vi "WriteOVABinFile.vi"(8 "error in (no error)":errorcluster, 10 "Matrix Selection":u8(ring) items=["A", "B", "C"], 11 "Measurement Data File Path":path) -> (0 "error out":errorcluster)   [LabVIEW 2012]
uses:
  bin/OVA32.dll
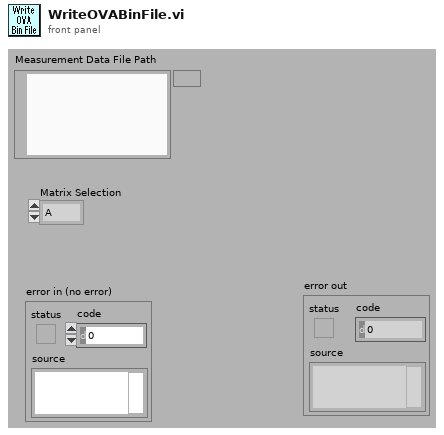
[diagram p1: front panel]
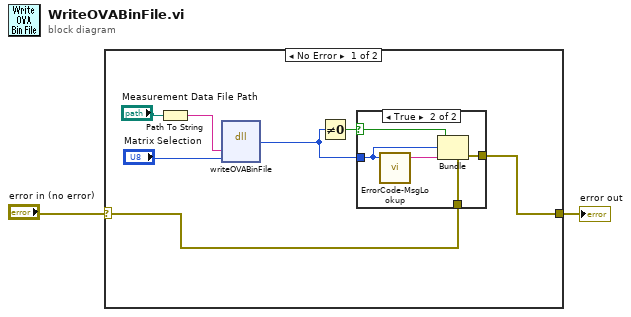
[diagram p0: block diagram]
diagram:
  n1 = case shown="No Error" "error in (no error)" {
    selector: "error in (no error)" -> [w7 w16]
    tunnel: [w6 w16] -> w1
    frame No Error {
      n2 = Path To String(path="Measurement Data File Path") -> (string=w3:string)
      n3 = dll-call lib="C:/_src/OVA5000_DSP_falcon/Software/LabVIEW/OVA/SDK/OVA_5000_SDK_v5.14.3/bin/OVA32.dll" fn="writeOVABinFile" label="writeOVABinFile()"("OVABinFileName"=w3, "measSelection"="Matrix Selection") -> (w8:i32)  [unwired: 5 in, 2 out]
      n4 = Not Equal To 0?(x=w8) -> (x != 0?=w9:bool)
      n5 = case shown="True" w9 {
        selector: w9 -> [_ w12]
        tunnel: w8 -> [_ w13]
        tunnel: w7 -> [w10 w15]
        tunnel: [w10 w11] -> w6
        frame False {
        }
        frame True {
          n6 = call "ErrorCode-MsgLookup.vi"("DLL Return Code"=w13) -> ("Error String"=w14:string)  [unwired: 2 in, 2 out]
          n7 = Bundle(cluster=w15, "status"=w12, "code"=w13, "source"=w14) -> (w11:errorcluster)
        }
      }
    }
    frame Error {
    }
  }
  "error out" <- w1
